vi "camera_asynchrone_acquisition.vi"() -> ()   [LabVIEW 2018]
uses:
  Controls/Image information.ctl
  Controls/Image general information.ctl
  Controls/Image acquisition information.ctl
  Controls/Point2D.ctl
  Controls/Data alignment enum.ctl
  Classes/Camera/Camera.lvclass
  Classes/CameraSet/CameraSet.lvclass
  Classes/Image/Image.lvclass
panel:
  out "Acquisition information":T1={"Image general information"={"Camera serial number"="", "Smearing removed"=FALSE, "Background image removed"=FALSE, "Time Stamp"=timestamp(0 s since 1904-01-01), "Comment"="", "Camera_MAX_Level"=0}, "Acquisition information"={"Exposure duration (us)"=0, "Exposure duration specified (us)"=0, "Gain"=0.0, "Number of summed images"=0, "Trigger type"=""}, "Number of pixels"={"X"=0, "Y"=0}, "Number of bits"=enum."16"}
  in  "Init":bool
  in  "Reset error":bool
  out "exposure_duration_us (get)":u32
  in  "exposure_duration_us (set)":u32=1000 min=1
  out "Current error":errorcluster
  out "nb_images (get)":u32=10
  in  "nb_images (set)":u32=1 min=1
  in  "Show camera signal":bool
  in  "Exit":bool
  in  "Stop Acq":bool
  in  "Start Acq":bool
  out "Image Camera":u32[][](graph)
  in  "Configuration file path":path
  # "Acquisition Parameters"
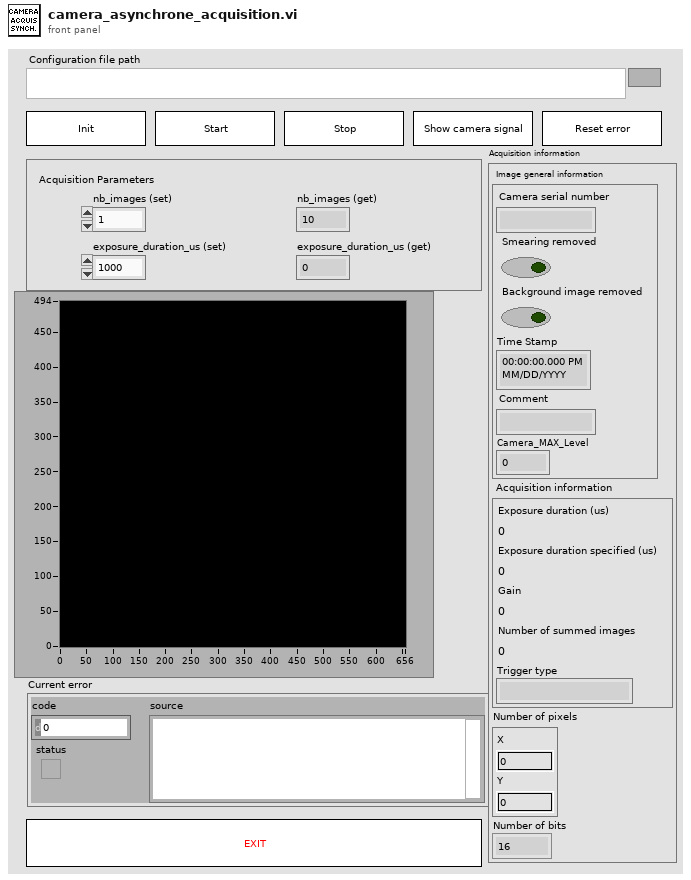
[diagram p1: front panel]
types:
  T1 = typedef "Image information.ctl" = cluster{"Image general information":T2, "Acquisition information":T3, "Number of pixels":T4, "Number of bits":T5}
  T2 = typedef "Image general information.ctl" = cluster{"Camera serial number":string, "Smearing removed":bool, "Background image removed":bool, "Time Stamp":timestamp, "Comment":string, "Camera_MAX_Level":i32}
  T3 = typedef "Image acquisition information.ctl" = cluster{"Exposure duration (us)":i32, "Exposure duration specified (us)":i32, "Gain":sgl, "Number of summed images":i32, "Trigger type":string}
  T4 = typedef "Point2D.ctl" = cluster{"X":u32, "Y":u32}
  T5 = typedef "Data alignment enum.ctl" = enum16{"8", "16", "32"}
  T6 = typedef "CameraSpecifications.ctl" = cluster{"Grabber name":string, "Camera name":string, "Camera sn":string, "Pixels_um":T7, "Maximum level":u32, "Data alignment":T5, "Is signed":bool, "Acquisition start":T4, "Acquisition length":T4, "MaxFrameRate_Hz":sgl, "Chip type":enum16{"Progressive scan", "Frame transfert"}}
  T7 = typedef "General dimensions definition.ctl" = cluster{"Size":T4, "Step":T8}
  T8 = typedef "Point2Df.ctl" = cluster{"X":sgl, "Y":sgl}
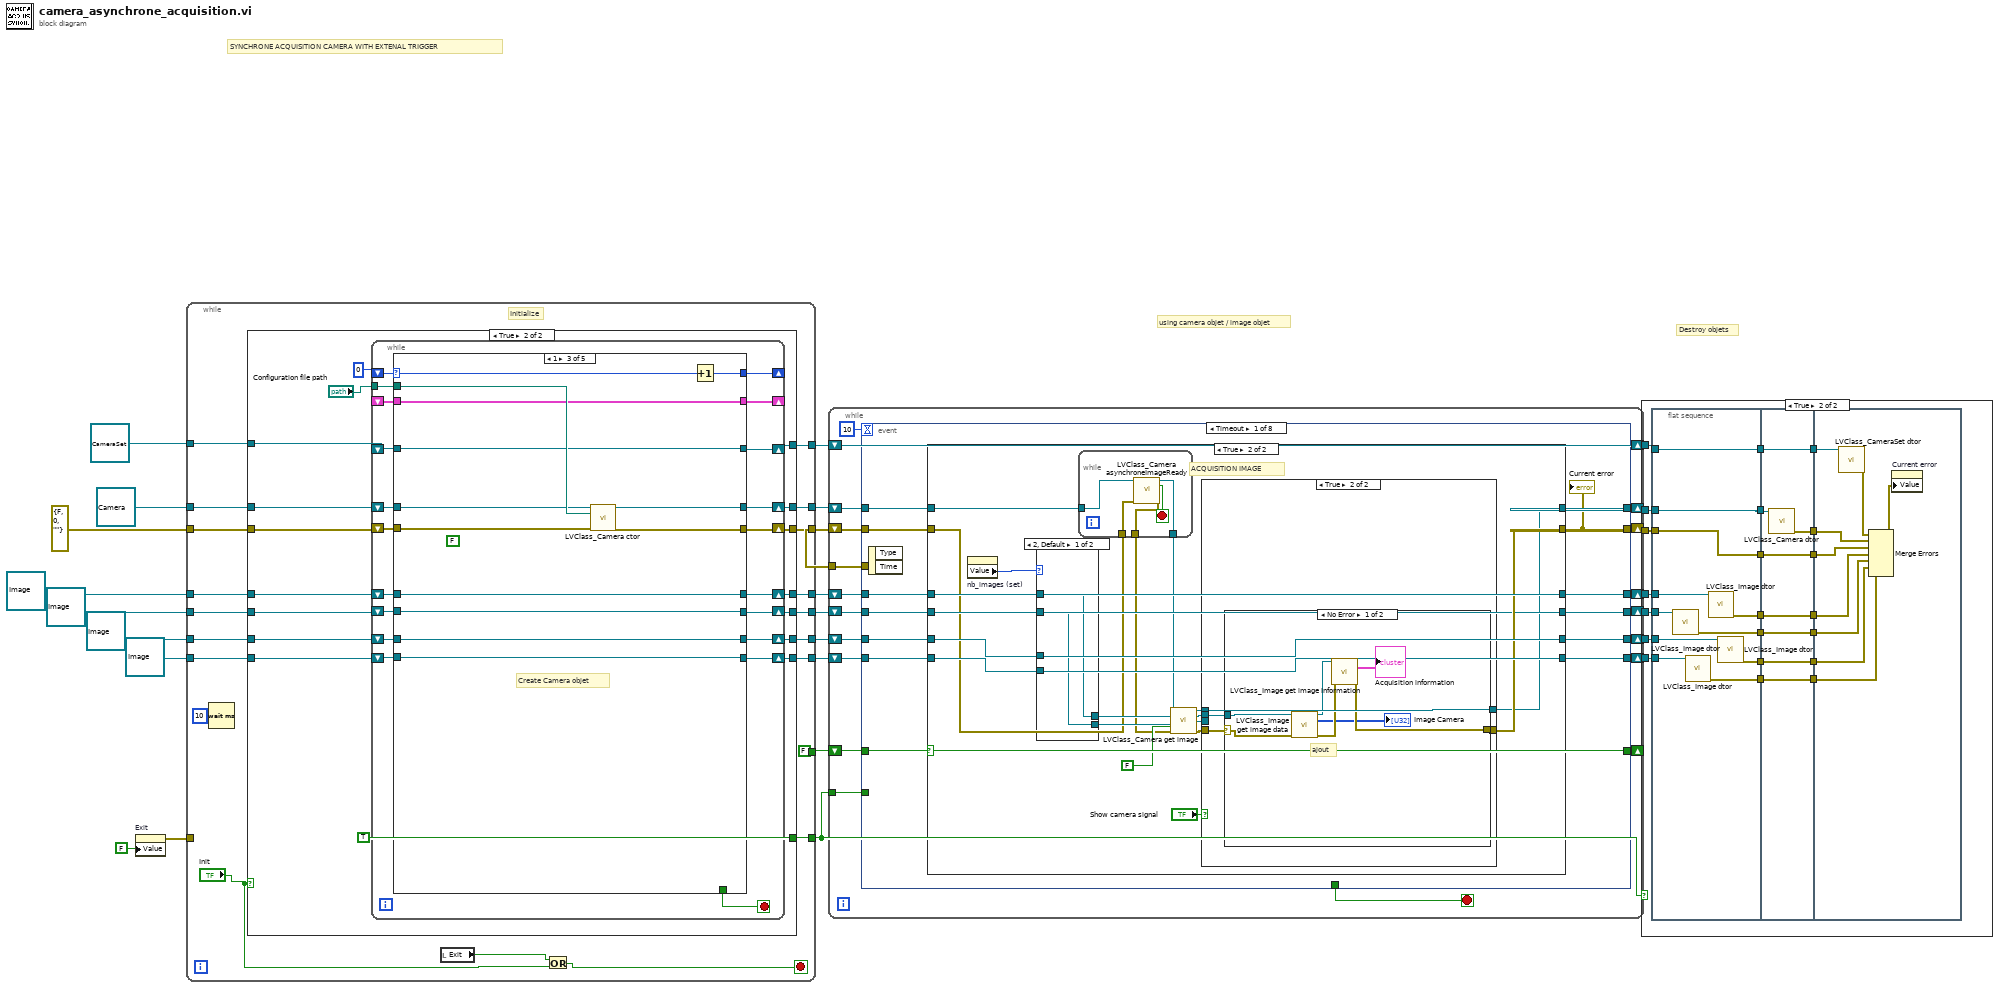
[diagram p0: block diagram]
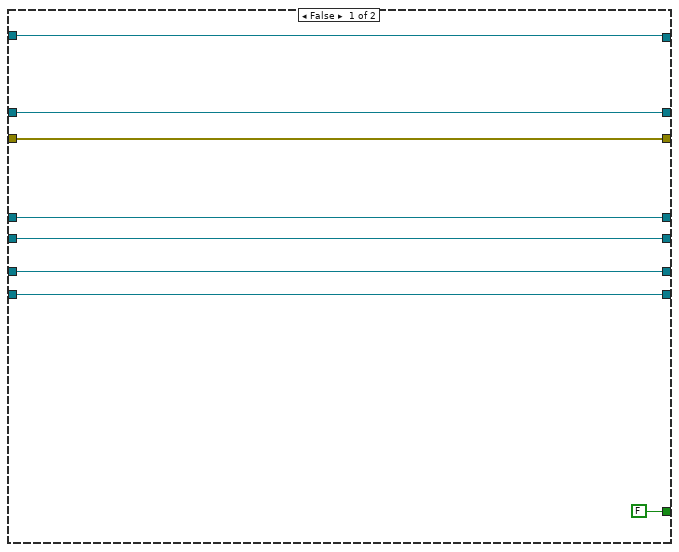
[diagram p3: hidden frame]
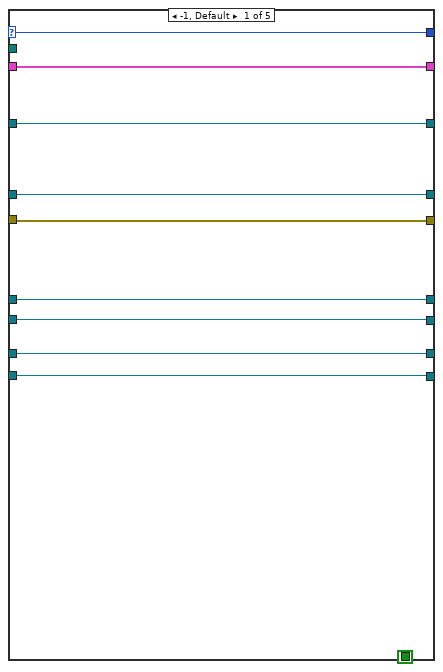
[diagram p4: hidden frame]
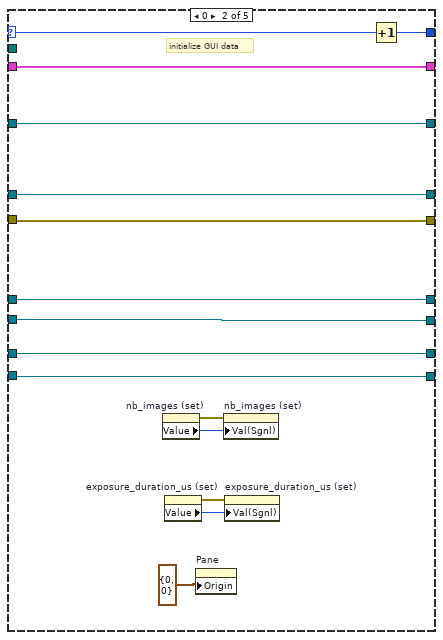
[diagram p5: hidden frame]
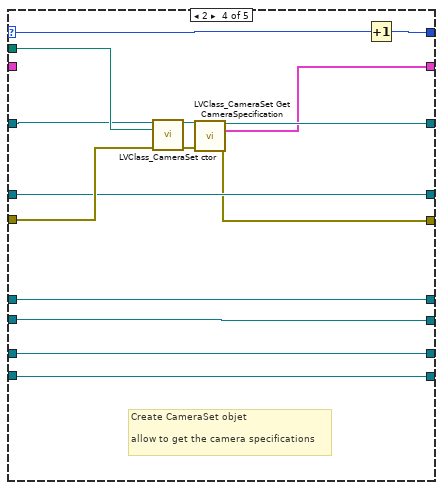
[diagram p6: hidden frame]
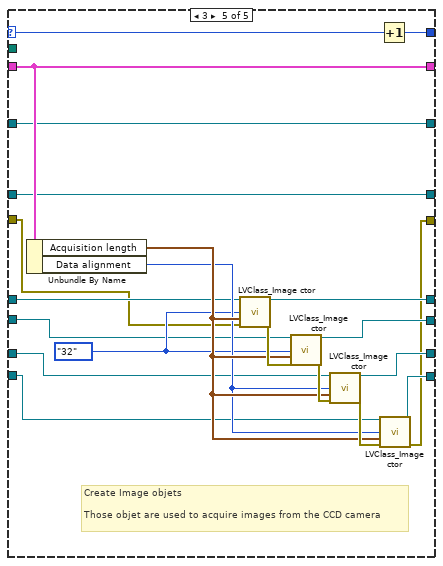
[diagram p7: hidden frame]
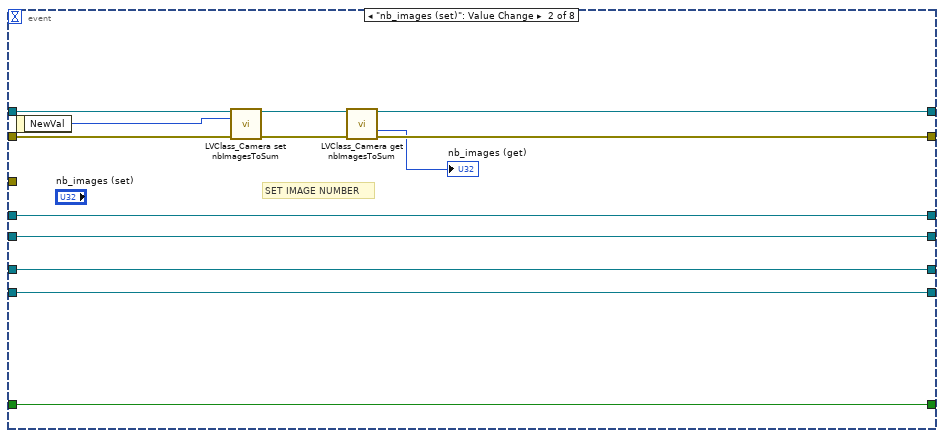
[diagram p12: hidden frame]
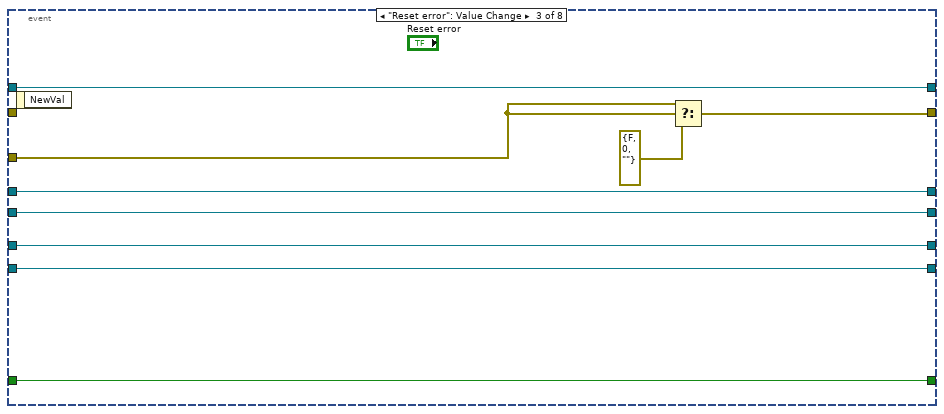
[diagram p13: hidden frame]
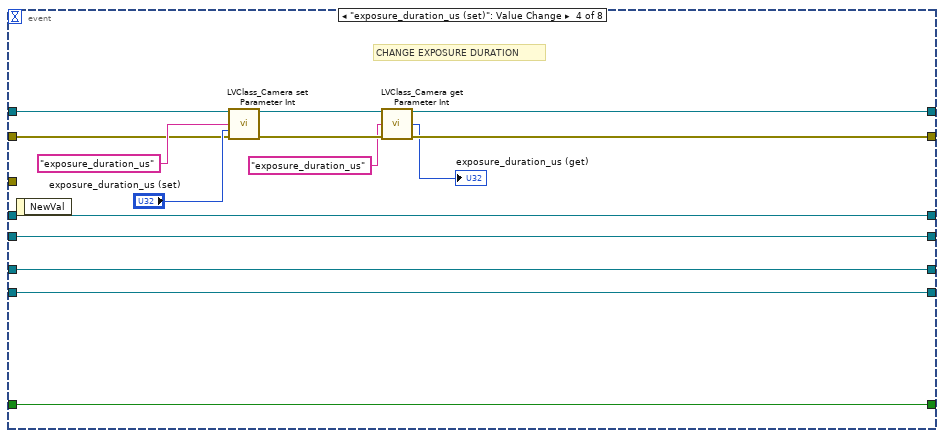
[diagram p14: hidden frame]
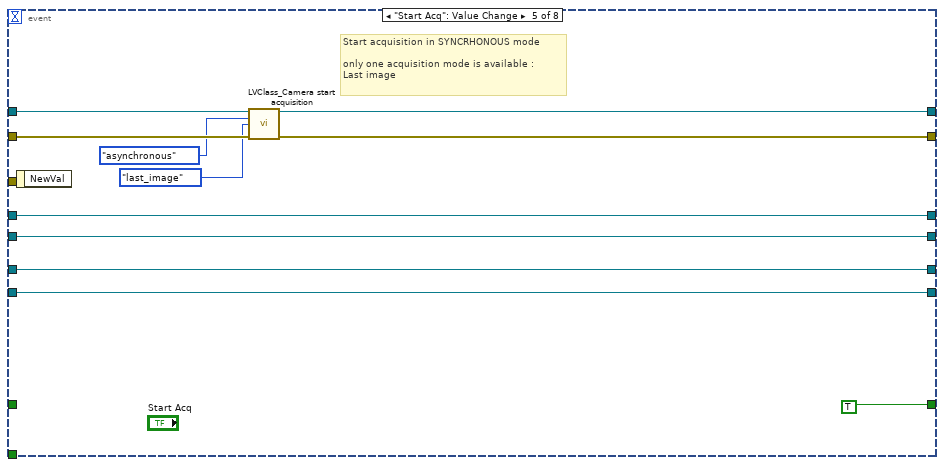
[diagram p15: hidden frame]
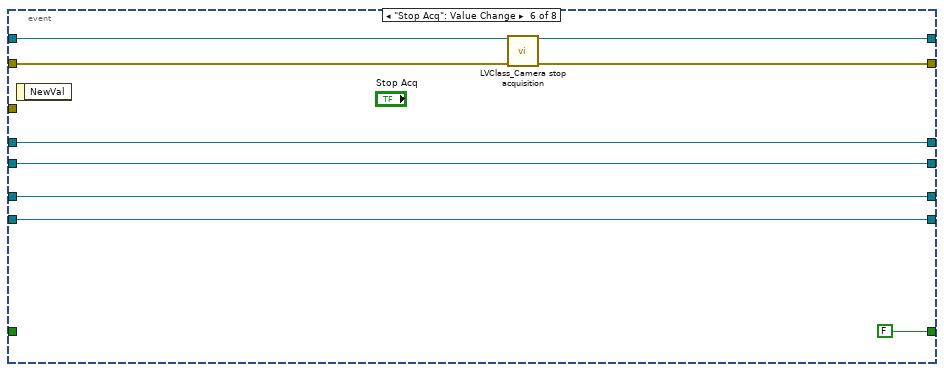
[diagram p16: hidden frame]
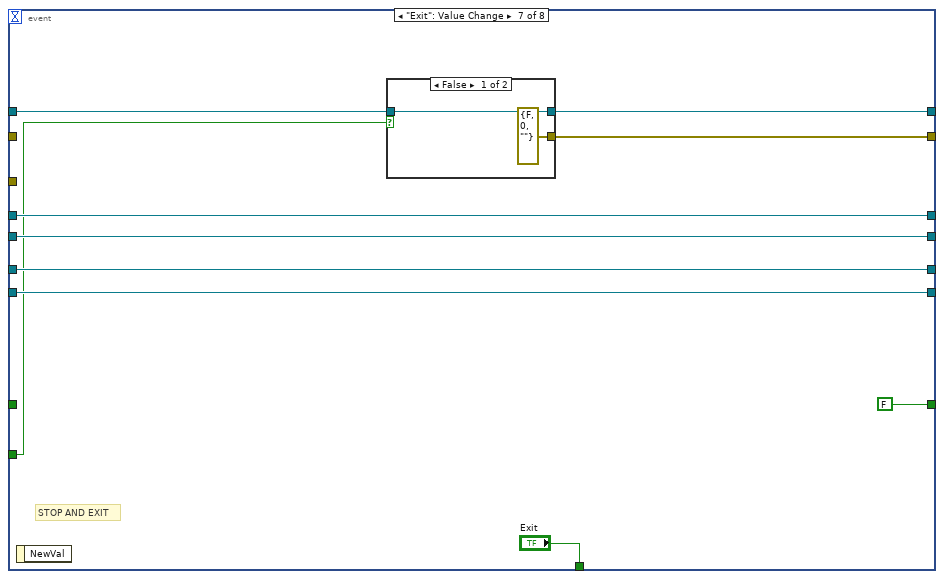
[diagram p17: hidden frame]
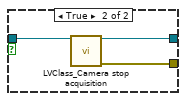
[diagram p18: hidden frame]
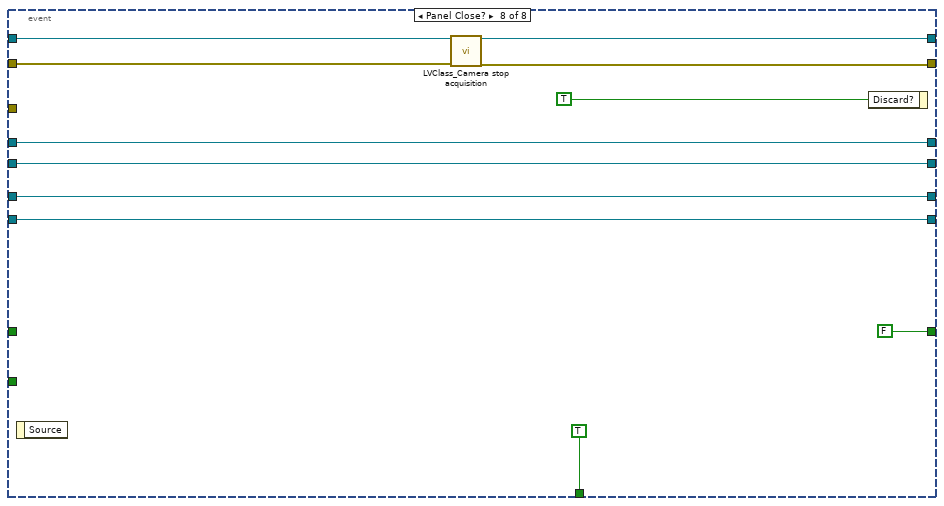
[diagram p19: hidden frame]
diagram:
  # "Destroy objets"
  # "using camera objet / image objet"
  # "SYNCHRONE ACQUISITION CAMERA WITH EXTENAL TRIGGER"
  n1 = property on="Exit" class="Bool (strict)"("Value"=FALSE ("Exit")) -> (error out=w1:errorcluster)  [unwired: 2 in, 1 out]
  n2 = while {
    tunnel: [FALSE] -> w18
    tunnel: [w44] -> w17
    tunnel: [w43] -> w16
    tunnel: [w42] -> w15
    tunnel: [w41] -> w14
    tunnel: [w40] -> w13
    tunnel: [w39] -> w12
    tunnel: refnum<class "Camera.lvclass"> refnum ("Camera.lvclass") -> [w38]
    tunnel: refnum<class "CameraSet.lvclass"> refnum ("CameraSet.lvclass") -> [w37]
    tunnel: refnum<class "Image.lvclass"> refnum ("Image in") -> [w36]
    tunnel: refnum<class "Image.lvclass"> refnum ("Image in") -> [w35]
    tunnel: refnum<class "Image.lvclass"> refnum ("Image in") -> [w34]
    tunnel: refnum<class "Image.lvclass"> refnum ("Image in") -> [w33]
    tunnel: errorcluster {"status"=FALSE, "code"=0, "source"=""} ("error out") -> [w32]
    tunnel: [w31] -> w4
    tunnel: [w29] -> w3
    tunnel: w1 -> [_]
    stop <- w26 stop-if-true
    # "Initialize"
    n3 = Wait (ms)(milliseconds to wait=u32 10) -> ()  [unwired: 1 out]
    n4 = case shown="True" "Init" {
      tunnel: [w53 w70] -> w44
      tunnel: [w52 w69] -> w43
      tunnel: [w50 w67] -> w42
      tunnel: [w49 w66] -> w41
      tunnel: [w48 w65] -> w40
      tunnel: [w47 w64] -> w39
      tunnel: w38 -> [w53 w63]
      tunnel: w37 -> [w52 w61]
      tunnel: w36 -> [w50 w60]
      tunnel: w35 -> [w49 w59]
      tunnel: w34 -> [w48 w58]
      tunnel: w33 -> [w47 w57]
      tunnel: w32 -> [w51 w56]
      tunnel: [w51 w55] -> w31
      tunnel: [FALSE TRUE] -> w29
      frame False {
      }
      frame True {
        n5 = while {
          tunnel: "Configuration file path" -> [w88]
          shift-right: [w90] -> w70
          shift-left: w63 -> [w82]
          shift-right: [w72] -> _
          shift-left: 0 -> [w71]
          shift-right: [w89] -> w69
          shift-left: w61 -> [w81]
          shift-right: [w80] -> _
          shift-left: _ -> [w78]
          shift-right: [w87] -> w67
          shift-left: w60 -> [w79]
          shift-right: [w86] -> w66
          shift-left: w59 -> [w77]
          shift-right: [w85] -> w65
          shift-left: w58 -> [w75]
          shift-right: [w84] -> w64
          shift-left: w57 -> [w76]
          shift-right: [w83] -> w55
          shift-left: w56 -> [w73]
          stop <- w74 stop-if-true
          n6 = case shown="1" w71 {
            tunnel: [w100 w102 w128 w136 w151] -> w90
            tunnel: w88 -> [_ _ w127 w140 _]
            tunnel: [w99 w106 w125 w141 w152] -> w89
            tunnel: [w92 w107 w119 w131 w158] -> w87
            tunnel: [w93 w108 w120 w132 w157] -> w86
            tunnel: [w94 w109 w121 w133 w156] -> w85
            tunnel: [w95 w110 w122 w134 w155] -> w84
            tunnel: [w96 w101 w124 w135 w154] -> w83
            selector: w71 -> [w91 w104 w117 w130 w146]
            tunnel: w82 -> [w100 w102 w126 w136 w151]
            tunnel: w81 -> [w99 w106 w125 w139 w152]
            tunnel: [w97 w103 w123 w138 w153] -> w80
            tunnel: w79 -> [w92 w107 w119 w131 w150]
            tunnel: w78 -> [w97 w103 w123 _ w153]
            tunnel: w77 -> [w93 w108 w120 w132 w149]
            tunnel: w76 -> [w95 w110 w122 w134 w148]
            tunnel: w75 -> [w94 w109 w121 w133 w147]
            tunnel: [TRUE _ _ _ _] -> w74
            tunnel: w73 -> [w96 w101 w116 w137 w144]
            tunnel: [w91 w105 w118 w129 w145] -> w72
            frame -1, Default {
            }
            frame 0 {
              # "initialize GUI data"
              n7 = property on="nb_images (set)" class="DigNum (strict)"() -> (error out=w115:errorcluster, "Value"=w114:u32)  [unwired: 2 in, 1 out]
              n8 = property on="exposure_duration_us (set)" class="DigNum (strict)"() -> (error out=w111:errorcluster, "Value"=w113:u32)  [unwired: 2 in, 1 out]
              n9 = property on="Pane" class="Pane"("Origin"=cluster{"Horizontal":i16, "Vertical":i16} {"Horizontal"=0, "Vertical"=0} ("Front Panel Window:Origin")) -> ()  [unwired: 2 in, 2 out]
              n10 = property on="nb_images (set)" class="DigNum (strict)"(error in=w115, "Val(Sgnl)"=w114) -> ()  [unwired: 1 in, 2 out]
              n11 = property on="exposure_duration_us (set)" class="DigNum (strict)"(error in=w111, "Val(Sgnl)"=w113) -> ()  [unwired: 1 in, 2 out]
              n12 = Increment(x=w104) -> (x+1=w105:i32)
            }
            frame 1 {
              (unwired) FALSE ("Acq required")
              # "Create Camera objet"
              n13 = call "LVClass_Camera ctor.vi"("Camera (const)"=w126, "Configuration file path"=w127, "error in (no error)"=w116) -> ("Camera (new)"=w128:refnum<class "Camera.lvclass">, "error out"=w124:errorcluster)  [unwired: 11 in]
              n14 = Increment(x=w117) -> (x+1=w118:i32)
            }
            frame 2 {
              # "Create CameraSet objet\n\nallow to get the camera specifications"
              n15 = call "LVClass_CameraSet ctor.vi"("CameraSet (const)"=w139, "Configuration file path"=w140, "error in (no error)"=w137) -> ("CameraSet (new)"=w143:refnum<class "CameraSet.lvclass">, "error out"=w142:errorcluster)  [unwired: 11 in]
              n16 = call "LVClass_CameraSet Get CameraSpecification.vi"("CameraSet in"=w143, "error in (no error)"=w142) -> ("CameraSet out"=w141:refnum<class "CameraSet.lvclass">, "Camera Config"=w138:T6, "error out"=w135:errorcluster)  [unwired: 11 in]
              n17 = Increment(x=w130) -> (x+1=w129:i32)
            }
            frame 3 {
              w159 = Data_alignment_enum."32" ("Data alignment")
              # "Create Image objets\n\nThose objet are used to acquire images from the CCD camera"
              n18 = Unbundle By Name(w153) -> ("Acquisition length"=w161:T4, "Data alignment"=w160:T5)
              n19 = call "LVClass_Image ctor.vi"("Image (const)"=w150, "Data alignment"=w159, "Size"=w161, "error in (no error)"=w144) -> ("Image (new)"=w158:refnum<class "Image.lvclass">, "error out"=w162:errorcluster)  [unwired: 10 in]
              n20 = call "LVClass_Image ctor.vi"("Image (const)"=w149, "Data alignment"=w159, "Size"=w161, "error in (no error)"=w162) -> ("Image (new)"=w157:refnum<class "Image.lvclass">, "error out"=w163:errorcluster)  [unwired: 10 in]
              n21 = call "LVClass_Image ctor.vi"("Image (const)"=w147, "Data alignment"=w160, "Size"=w161, "error in (no error)"=w163) -> ("Image (new)"=w156:refnum<class "Image.lvclass">, "error out"=w164:errorcluster)  [unwired: 10 in]
              n22 = Increment(x=w146) -> (x+1=w145:i32)
              n23 = call "LVClass_Image ctor.vi"("Image (const)"=w148, "Data alignment"=w160, "Size"=w161, "error in (no error)"=w164) -> ("Image (new)"=w155:refnum<class "Image.lvclass">, "error out"=w154:errorcluster)  [unwired: 10 in]
            }
          }
        }
      }
    }
    n24 = local read "Exit"() -> (w28:bool)
    n25 = Or(x=w28, y="Init") -> (x .or. y?=w26:bool)
  }
  n26 = while {
    shift-right: [w180] -> w25
    shift-left: w4 -> [w182]
    shift-right: [w178] -> w24
    shift-left: w17 -> [w179]
    shift-right: [w172] -> w23
    shift-left: w15 -> [w177]
    shift-right: [w171] -> w22
    shift-left: w14 -> [w176]
    shift-right: [w170] -> w21
    shift-left: w13 -> [w175]
    shift-right: [w169] -> w20
    shift-left: w12 -> [w174]
    shift-right: [w168] -> _
    shift-left: w18 -> [w173]
    shift-right: [w167] -> w19
    shift-left: w16 -> [w167]
    tunnel: w4 -> [w166]
    tunnel: w3 -> [w165]
    stop <- w181 stop-if-true
    n27 = event shown="[0] Timeout" {
      selector: _ -> [_ _ _ _ _ _ _ _]
      dyn-events: _ -> [_ _ _ _ _ _ _ _]
      timeout: 10 -> [_ _ _ _ _ _ _ _]
      tunnel: w182 -> [w188 w256 _ w279 w291 w293 _ w318]
      tunnel: [_ _ _ _ _ _ "Exit" TRUE ("Exit")] -> w181
      tunnel: [w184 w254 w259 w274 w289 w299 w309 w323] -> w180
      tunnel: w179 -> [w193 w255 w261 w278 w292 w300 w310 w325]
      tunnel: [w192 w253 w261 w275 w290 w301 w308 w324] -> w178
      tunnel: w177 -> [w196 w246 w263 w268 w286 w295 w304 w319]
      tunnel: w176 -> [w195 w247 w264 w269 w285 w296 w305 w320]
      tunnel: w175 -> [w194 w248 w265 w270 w284 w297 w306 w321]
      tunnel: w174 -> [w189 w249 w266 w271 w283 w298 w307 w322]
      tunnel: w173 -> [w185 w245 w262 w267 _ _ _ _]
      tunnel: [w191 w246 w263 w268 w286 w295 w304 w319] -> w172
      tunnel: [w190 w247 w264 w269 w285 w296 w305 w320] -> w171
      tunnel: [w187 w248 w265 w270 w284 w297 w306 w321] -> w170
      tunnel: [w186 w249 w266 w271 w283 w298 w307 w322] -> w169
      tunnel: [w185 w245 w262 w267 TRUE FALSE FALSE FALSE] -> w168
      tunnel: w166 -> [_ _ w258 _ _ _ _ _]
      tunnel: w165 -> [_ _ _ _ _ _ w302 _]
      event Timeout {
        n28 = event-data() -> ()  [unwired: 1 in, 2 out]
        n29 = case shown="True" w185 {
          tunnel: [w197 w211] -> w184
          tunnel: w196 -> [w202 w217]
          tunnel: [w202 w217] -> w191
          tunnel: [w198 w208] -> w190
          tunnel: w194 -> [w201 w216]
          tunnel: w189 -> [w200 w215]
          tunnel: [w201 w216] -> w187
          tunnel: [w200 w215] -> w186
          tunnel: w195 -> [w198 w208]
          tunnel: w193 -> [w199 w206]
          tunnel: [w199 w207] -> w192
          tunnel: w188 -> [w197 w204]
          frame False {
          }
          frame True {
            # "ACQUISITION IMAGE"
            n30 = property on="nb_images (set)" class="DigNum (strict)"() -> ("Value"=w218:u32)  [unwired: 2 in, 2 out]
            n31 = case shown="2, Default" w218 {
              tunnel: [w228 w230] -> w219
              tunnel: w208 -> [w227 _]
              tunnel: w217 -> [w228 _]
              tunnel: [w227 w229] -> w214
              tunnel: w216 -> [_ w230]
              tunnel: w215 -> [_ w229]
              frame 2, Default {
              }
              frame 1 {
              }
            }
            n32 = while {
              tunnel: w206 -> [w226]
              tunnel: [w225] -> w205
              tunnel: w204 -> [w223]
              tunnel: [w222] -> w203
              stop <- w224 stop-if-true
              n33 = call "LVClass_Camera asynchroneImageReady.vi"("Camera in"=w226, "error in (no error)"=w223) -> ("Camera out"=w225:refnum<class "Camera.lvclass">, "ready"=w224:bool, "error out"=w222:errorcluster)  [unwired: 11 in]
            }
            n34 = call "LVClass_Camera get image.vi"("Camera in"=w205, "Image"=w219, "Image RAW"=w214, "remove_background"=FALSE, "error in (no error)"=w203) -> ("Camera out"=w221:refnum<class "Camera.lvclass">, "Image (dup)"=w212:refnum<class "Image.lvclass">, "Image (dup) RAW"=w213:refnum<class "Image.lvclass">, "error out"=w209:errorcluster)  [unwired: 7 in]
            n35 = case shown="True" "Show camera signal" {
              tunnel: w221 -> [w232 w233]
              tunnel: w212 -> [_ w234]
              tunnel: w209 -> [w231 w236]
              tunnel: [w232 w233] -> w207
              tunnel: [w231 w235] -> w211
              tunnel: w213 -> [_ _]
              frame False {
              }
              frame True {
                n36 = case shown="No Error" w236 {
                  selector: w236 -> [w243 w244]
                  tunnel: [w240 w244] -> w235
                  tunnel: w234 -> [w239 _]
                  frame No Error {
                    # "ajout"
                    n37 = call "LVClass_Image get image data.vi"("Image in"=w239, "error in (no error)"=w243) -> ("Image out"=w242:refnum<class "Image.lvclass">, "Image data out"=→"Image Camera":u32[][], "error out"=w241:errorcluster)  [unwired: 11 in]
                    n38 = call "LVClass_Image get image information.vi"("Image in"=w242, "error in (no error)"=w241) -> ("Acquisition information"=→"Acquisition information":T1, "error out"=w240:errorcluster)  [unwired: 11 in, 1 out]
                  }
                  frame Error {
                  }
                }
              }
            }
          }
        }
        "Current error" <- w184
      }
      event "nb_images (set)": Value Change {
        # "SET IMAGE NUMBER"
        n39 = event-data() -> ("NewVal"=w257:u32)  [unwired: 1 in]
        n40 = call "LVClass_Camera set nbImagesToSum.vi"("Camera in"=w255, "nb_image"=w257, "error in (no error)"=w256) -> ("Camera out"=w252:refnum<class "Camera.lvclass">, "error out"=w251:errorcluster)  [unwired: 11 in]
        n41 = call "LVClass_Camera get nbImagesToSum.vi"("Camera in"=w252, "error in (no error)"=w251) -> ("Camera out"=w253:refnum<class "Camera.lvclass">, "nb_image"=→"nb_images (get)":u32, "error out"=w254:errorcluster)  [unwired: 11 in]
      }
      event "Reset error": Value Change {
        n42 = event-data() -> ()  [unwired: 1 in, 1 out]
        n43 = Select(t=w258, s=w258, f=errorcluster {"status"=FALSE, "code"=0, "source"=""} ("error out")) -> (s? t:f=w259:errorcluster)
      }
      event "exposure_duration_us (set)": Value Change {
        # "CHANGE EXPOSURE DURATION"
        n44 = event-data() -> ()  [unwired: 1 in, 1 out]
        n45 = call "LVClass_Camera set Parameter Int.vi"("Camera in"=w278, "parameter_name"="exposure_duration_us", "value"="exposure_duration_us (set)", "error in (no error)"=w279) -> ("Camera out"=w277:refnum<class "Camera.lvclass">, "error out"=w276:errorcluster)  [unwired: 10 in]
        n46 = call "LVClass_Camera get Parameter Int.vi"("Camera in"=w277, "parameter_name"="exposure_duration_us", "error in (no error)"=w276) -> ("Camera out"=w275:refnum<class "Camera.lvclass">, "value"=→"exposure_duration_us (get)":i32, "error out"=w274:errorcluster)  [unwired: 10 in]
      }
      event "Start Acq": Value Change {
        # "Start acquisition in SYNCRHONOUS mode\n\nonly one acquisition mode is available :\nLast image"
        n47 = event-data() -> ()  [unwired: 1 in, 1 out]
        n48 = call "LVClass_Camera start acquisition.vi"("Camera in"=w292, "synchronisation_mode"=enum16{"synchronous", "asynchronous"}."asynchronous", "acquisition_mode"=enum16{"last_image", "new_image"}."last_image", "error in (no error)"=w291) -> ("Camera out"=w290:refnum<class "Camera.lvclass">, "error out"=w289:errorcluster)  [unwired: 10 in]
      }
      event "Stop Acq": Value Change {
        n49 = event-data() -> ()  [unwired: 1 in, 1 out]
        n50 = call "LVClass_Camera stop acquisition.vi"("Camera in"=w300, "error in (no error)"=w293) -> ("Camera out"=w301:refnum<class "Camera.lvclass">, "error out"=w299:errorcluster)  [unwired: 12 in]
      }
      event "Exit": Value Change {
        # "STOP AND EXIT"
        n51 = event-data() -> ()  [unwired: 1 in, 1 out]
        n52 = case shown="False" w302 {
          tunnel: w310 -> [w313 w316]
          tunnel: [errorcluster {"status"=FALSE, "code"=0, "source"=""} ("error out") w315] -> w309
          tunnel: [w313 w314] -> w308
          frame False {
          }
          frame True {
            n53 = call "LVClass_Camera stop acquisition.vi"("Camera in"=w316) -> ("Camera out"=w314:refnum<class "Camera.lvclass">, "error out"=w315:errorcluster)  [unwired: 13 in]
          }
        }
      }
      event Panel Close? {
        n54 = event-data() -> ()  [unwired: 1 in, 1 out]
        n55 = call "LVClass_Camera stop acquisition.vi"("Camera in"=w325, "error in (no error)"=w318) -> ("Camera out"=w324:refnum<class "Camera.lvclass">, "error out"=w323:errorcluster)  [unwired: 12 in]
        n56 = event-data("Discard?"=TRUE) -> ()  [unwired: 1 in, 1 out]
      }
    }
  }
  n57 = case shown="True" w3 {
    tunnel: w25 -> [_ w334]
    tunnel: w24 -> [_ w333]
    tunnel: w23 -> [_ w332]
    tunnel: w22 -> [_ w331]
    tunnel: w21 -> [_ w330]
    tunnel: w20 -> [_ w329]
    tunnel: w19 -> [_ w328]
    frame False {
    }
    frame True {
      n58 = flat-sequence {
        tunnel: w333 -> [w359]
        tunnel: w334 -> [w357]
        tunnel: [w359] -> w348
        tunnel: w328 -> [w358]
        tunnel: [w358] -> w347
        tunnel: [w357] -> w346
        tunnel: w332 -> [w356]
        tunnel: w331 -> [w355]
        tunnel: w330 -> [w354]
        tunnel: w329 -> [w353]
        tunnel: [w352] -> w345
        tunnel: [w351] -> w344
        tunnel: [w350] -> w343
        tunnel: [w349] -> w342
        tunnel: w348 -> [w367]
        tunnel: w347 -> [w366]
        tunnel: w346 -> [w364]
        tunnel: [w366] -> w341
        tunnel: [w365] -> w340
        tunnel: [w364] -> w339
        tunnel: w345 -> [w363]
        tunnel: [w363] -> w338
        tunnel: w344 -> [w362]
        tunnel: [w362] -> w337
        tunnel: w343 -> [w361]
        tunnel: [w361] -> w336
        tunnel: w342 -> [w360]
        tunnel: [w360] -> w335
        tunnel: w341 -> [w376]
        tunnel: w340 -> [w374]
        tunnel: w339 -> [w373]
        tunnel: w338 -> [w372]
        tunnel: w337 -> [w371]
        tunnel: w336 -> [w370]
        tunnel: w335 -> [w369]
        frame #0 {
          n59 = call "LVClass_Image dtor.vi"("Image in"=w355) -> ("error out"=w351:errorcluster)  [unwired: 13 in, 1 out]
          n60 = call "LVClass_Image dtor.vi"("Image in"=w353) -> ("error out"=w349:errorcluster)  [unwired: 13 in, 1 out]
          n61 = call "LVClass_Image dtor.vi"("Image in"=w356) -> ("error out"=w352:errorcluster)  [unwired: 13 in, 1 out]
          n62 = call "LVClass_Image dtor.vi"("Image in"=w354) -> ("error out"=w350:errorcluster)  [unwired: 13 in, 1 out]
        }
        frame #1 {
          n63 = call "LVClass_Camera dtor.vi"("Camera in"=w367) -> ("error out"=w365:errorcluster)  [unwired: 13 in, 1 out]
        }
        frame #2 {
          n64 = call "LVClass_CameraSet dtor.vi"("CameraSet in"=w376) -> ("error out"=w375:errorcluster)  [unwired: 13 in, 1 out]
          n65 = Merge Errors(w375, w374, w373, w372, w371, w370, w369) -> (w368:errorcluster)
          n66 = property on="Current error" class="Clust (strict)"("Value"=w368) -> ()  [unwired: 2 in, 2 out]
        }
      }
    }
  }
